vi "set_com_port.vi"(8 "error in (no error)":errorcluster, 11 "LightSourceMH110125Tsunami in":refnum<class "LightSourceMH110125Tsunami.lvclass">) -> (0 "error out":errorcluster, 3 "LightSourceMH110125Tsunami out":refnum<class "LightSourceMH110125Tsunami.lvclass">)   [LabVIEW 2010, in "LightSourceMH110125Tsunami.lvclass"]
uses:
  LightSourceMH110125Tsunami.lvclass
  LightSourceMH110125Tsunami.lvclass/LightSourceMH110125Tsunami.ctl
panel:
  in  "comm port":refnum<visa-resource-name>
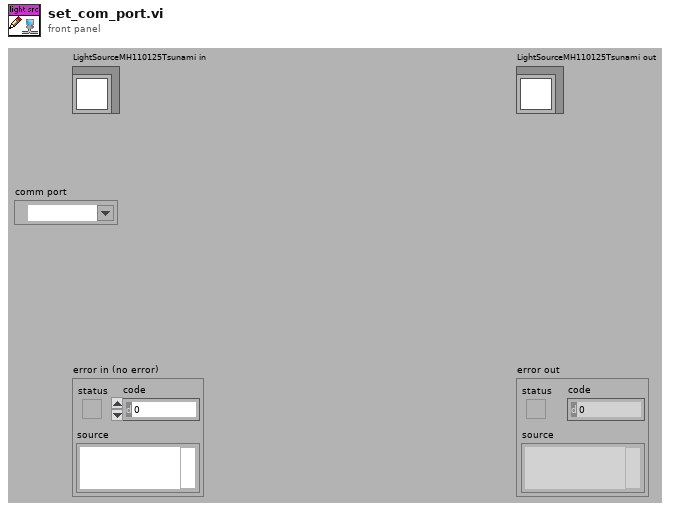
[diagram p1: front panel]
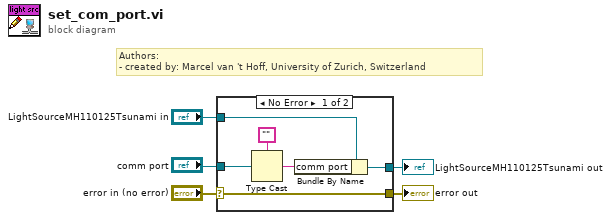
[diagram p0: block diagram]
diagram:
  # "Authors: \n- created by: Marcel van 't Hoff, University of Zurich, Switzerland"
  n1 = case shown="No Error" "error in (no error)" {
    selector: "error in (no error)" -> [w11 w12]
    tunnel: [w11 w12] -> w4
    tunnel: [w9 w13] -> w2
    tunnel: "LightSourceMH110125Tsunami in" -> [w10 w13]
    tunnel: "comm port" -> [w7 _]
    frame No Error {
      n2 = Type Cast(type="", x=w7) -> (*(type *) &x=w6:string)
      n3 = Bundle By Name(cluster=w10, "comm port"=w6) -> (w9:refnum<class "LightSourceMH110125Tsunami.lvclass">)
    }
    frame Error {
    }
  }
  "error out" <- w4
  "LightSourceMH110125Tsunami out" <- w2
